vi "Read Parameter.vi"(6 "value byte count":u8(ring) items=["variable"=0, "1"=1, "2"=2, "4"=4], 7 "process number":u8=1, 8 "error in (no error)":errorcluster, 9 "parameter number":u8, 10 "node address (same)":u8, 11 "ProPar in":refnum<class "PL Bronkhorst ProPar.lvclass">) -> (0 "error out":errorcluster, 2 "value":u8[](array[numeric]), 3 "ProPar out":refnum<class "PL Bronkhorst ProPar.lvclass">)   [LabVIEW 2015, in "PL Bronkhorst ProPar.lvclass"]
doc: "Read specified <b>parameter</b> of the specified <b>node</b>."
uses:
  PL Bronkhorst ProPar.lvclass
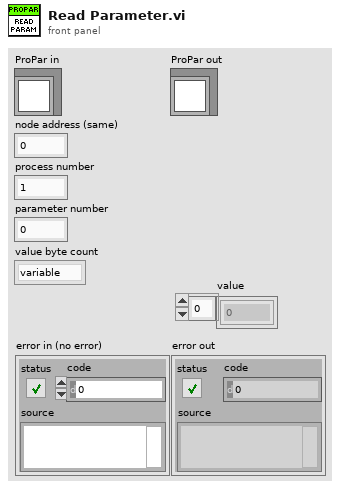
[diagram p1: front panel]
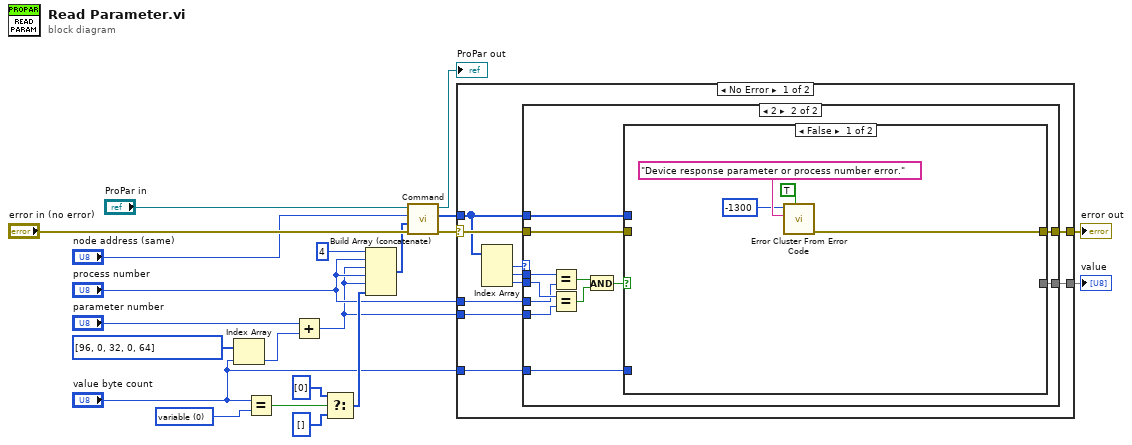
[diagram p0: block diagram]
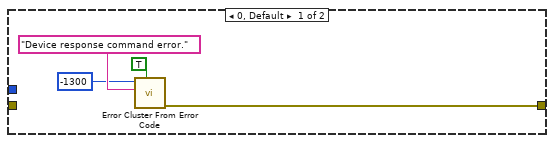
[diagram p2: hidden frame]
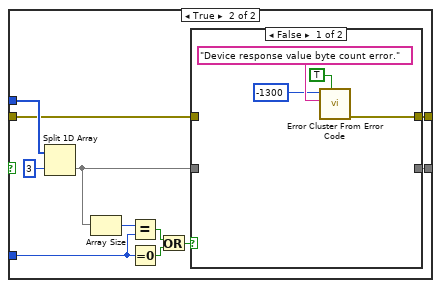
[diagram p3: hidden frame]
diagram:
  w3 = u8 0 items=["variable"=0, "1"=1, "2"=2, "4"=4] ("value byte count (variable) 2")
  n1 = Index Array(array=u8[] [96, 0, 32, 0, 64], index="value byte count") -> (element=w4:u8)
  n2 = Equal?(x="value byte count", y=w3) -> (x = y?=w2:bool)
  n3 = Add(x="parameter number", y=w4) -> (x+y=w7:u8)
  n4 = Select(t=u8[] [0] ("appended array"), s=w2, f=u8[] [] ("appended array")) -> (s? t:f=w9:u8[])
  n5 = Build Array (concatenate)(u8 4 ("node"), "process number", w7, "process number", w7, w9) -> (w15:u8[])
  n6 = call "Command.vi"("error in (no error)"="error in (no error)", "command data"=w15, "node address"="node address (same)", "ProPar in"="ProPar in") -> ("error out"=w14:errorcluster, "response data"=w12:u8[], "ProPar out"=→"ProPar out":refnum<class "PL Bronkhorst ProPar.lvclass">)  [unwired: 5 in]
  n7 = case shown="No Error" w14 {
    selector: w14 -> [w30 w69]
    tunnel: [w31 w69] -> w13
    tunnel: w12 -> [w28 _]
    tunnel: "process number" -> [w25 _]
    tunnel: w7 -> [w24 _]
    tunnel: [w23 _] -> w6
    tunnel: "value byte count" -> [w22 _]
    frame No Error {
      n8 = Index Array(array=w28) -> (element #1=w29:u8, element #2=w27:u8, element #3=w26:u8)  [unwired: 3 in]
      n9 = case shown="2" w29 {
        tunnel: [w32 w39] -> w31
        tunnel: w30 -> [_ w40]
        tunnel: w28 -> [_ w38]
        tunnel: w27 -> [_ w46]
        tunnel: w26 -> [_ w47]
        tunnel: w25 -> [_ w45]
        tunnel: w24 -> [_ w44]
        tunnel: [_ w37] -> w23
        tunnel: w22 -> [_ w36]
        frame 0, Default {
          n10 = call <vilib>:"Error Cluster From Error Code.vi"("show call chain? (False)"=TRUE, "error message (\"\")"="Device response command error." ("format string"), "error code (0)"=-1300) -> ("error out"=w32:errorcluster)  [unwired: 6 in]
        }
        frame 2 {
          n11 = Equal?(x=w46, y=w45) -> (x = y?=w43:bool)
          n12 = Equal?(x=w47, y=w44) -> (x = y?=w42:bool)
          n13 = And(x=w43, y=w42) -> (x .and. y?=w41:bool)
          n14 = case shown="False" w41 {
            tunnel: w40 -> [_ w53]
            tunnel: [w48 w52] -> w39
            tunnel: w38 -> [_ w62]
            tunnel: [_ w54] -> w37
            tunnel: w36 -> [_ w60]
            frame False {
              n15 = call <vilib>:"Error Cluster From Error Code.vi"("show call chain? (False)"=TRUE, "error message (\"\")"="Device response parameter or process number error." ("format string"), "error code (0)"=-1300) -> ("error out"=w48:errorcluster)  [unwired: 6 in]
            }
            frame True {
              n16 = Split 1D Array(array=w62, index=3) -> (second subarray=w55:u8[])  [unwired: 1 out]
              n17 = Array Size(array=w55) -> (size(s)=w59:i32)
              n18 = Equal?(x=w59, y=w60) -> (x = y?=w57:bool)
              n19 = Equal To 0?(x=w60) -> (x = 0?=w58:bool)
              n20 = Or(x=w57, y=w58) -> (x .or. y?=w56:bool)
              n21 = case shown="False" w56 {
                tunnel: w55 -> [_ w68]
                tunnel: [_ w68] -> w54
                tunnel: w53 -> [_ w67]
                tunnel: [w63 w67] -> w52
                frame False {
                  n22 = call <vilib>:"Error Cluster From Error Code.vi"("show call chain? (False)"=TRUE, "error message (\"\")"="Device response value byte count error." ("format string"), "error code (0)"=-1300) -> ("error out"=w63:errorcluster)  [unwired: 6 in]
                }
                frame True {
                }
              }
            }
          }
        }
      }
    }
    frame Error {
    }
  }
  "error out" <- w13
  "value" <- w6
